vi "Render Glyph.vi"(8 "error in (no error)":errorcluster, 11 "glyph slot":i64) -> (0 "error out":errorcluster, 3 "glyph slot 2":i64)   [LabVIEW 2023, in "Freetype Drawer.lvlib"]
uses:
  Freetype Drawer.lvlib
  libfreetype.dll
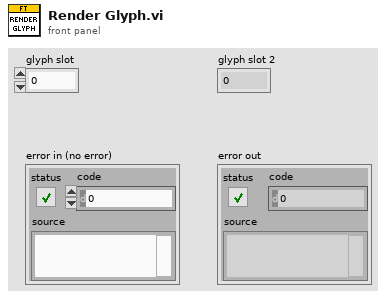
[diagram p1: front panel]
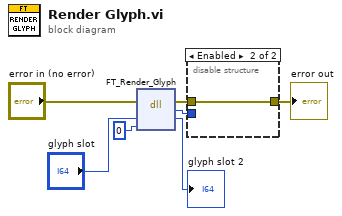
[diagram p0: block diagram]
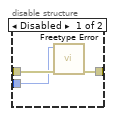
[diagram p2: hidden frame]
diagram:
  n1 = dll-call lib="E:/Labview/LV 2023/Libs/LV Symbol/Freetype Drawer/Wrappers/libfreetype.dll" fn="FT_Render_Glyph"(error in="error in (no error)", "glyph slot"="glyph slot", "render_mode"=0) -> (error out=w6:errorcluster, "error"=w5:i32, "glyph slot"=→"glyph slot 2":i64)  [unwired: 3 in, 1 out]
  n2 = disable-structure shown="Enabled" {
    disable-tunnel: w6 -> [w10 w11]
    disable-tunnel: w5 -> [w9 _]
    disable-tunnel: [w8 w11] -> w4
    frame Disabled {
      n3 = call "Freetype Error.vi"("error in (no error)"=w10, "Error"=w9) -> ("error out"=w8:errorcluster)  [unwired: 9 in]
    }
    frame Enabled {
    }
  }
  "error out" <- w4
